vi "Data_GetAcqTimestamp.vi"(8 "error in (no error)":errorcluster, 11 "data":variant) -> (0 "error out":errorcluster, 1 "timestamp":string, 2 "timestamp":timestamp, 3 "data out":variant)   [LabVIEW 2017, in "FileManager.lvlib"]
uses:
  <vilib>/addons/InsightCM/Devices/Shared/Common/FileManager/FileManager.lvlib
  <vilib>/addons/InsightCM/Devices/Shared/Common/FileManager/controls/DataPropertyNames.ctl
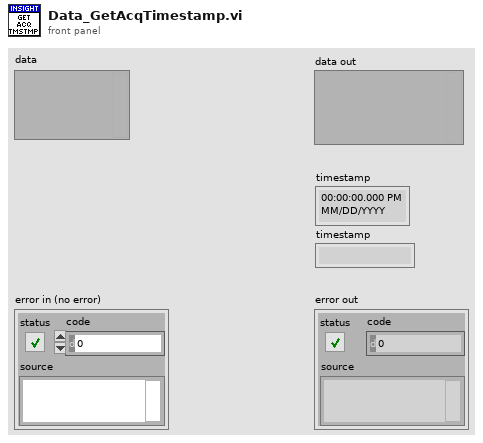
[diagram p1: front panel]
types:
  T1 = typedef "DataPropertyNames.ctl" = enum16{"Type", "EventRef", "FilePath", "DataGroup", "AcquisitionTimestamp", "StreamId", "StreamBlock", "TrendPointsOnly", "ExtraLargeFile"}
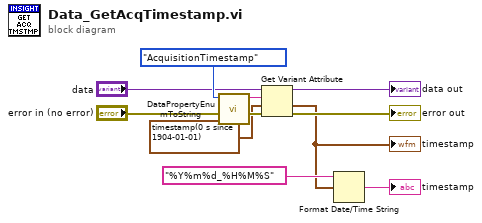
[diagram p0: block diagram]
diagram:
  n1 = call <vilib>:"DataPropertyEnumToString.vi"("property"=DataPropertyNames."AcquisitionTimestamp" ("Names")) -> ("string"=w10:string)  [unwired: 10 in]
  n2 = Get Variant Attribute(Variant="data", name=w10, default value (empty Variant)=timestamp(0 s since 1904-01-01) ("Time Stamp out"), error in="error in (no error)") -> (duplicate Variant=→"data out":variant, value=w2:timestamp, error out=→"error out":errorcluster)  [unwired: 1 out]
  "timestamp" <- w2
  n3 = Format Date/Time String(time format string (%c)="%Y%m%d_%H%M%S", seconds (now)=w2) -> (date/time string=→"timestamp":string)  [unwired: 1 in]
